vi "Value.vi"(7 "Variables":refnum<class "Variables.lvclass">, 11 "Condition Value in":refnum<class "Condition Value.lvclass">) -> (2 "error out":errorcluster, 3 "Value":dbl)   [LabVIEW 2020, in "VolatusSeq.lvlib" / "Condition Value.lvclass"]
uses:
  Condition Value.lvclass
  Variables/Variables.lvclass
  Condition Value.lvclass/Condition Value.ctl
  lv-vecto/Vecto/Channel DBL/Channel DBL.lvclass/Channel DBL.ctl
  Variables/Variables.lvclass/Variables.ctl
  lv-vecto/Vecto/Group DBL/Value by Index.vi
  lv-vecto/Vecto/Channel DBL/Channel DBL.lvclass
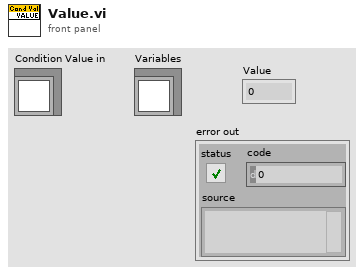
[diagram p1: front panel]
types:
  T1 = typedef "VolatusSeq.lvlib/Value Source.ctl" = enum16{"Channel", "Variable", "Expression"}
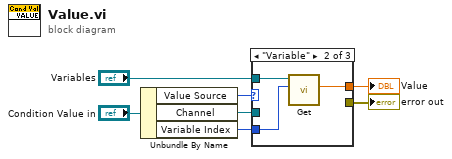
[diagram p0: block diagram]
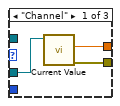
[diagram p2: hidden frame]
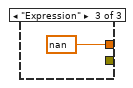
[diagram p3: hidden frame]
diagram:
  n1 = Unbundle By Name("Condition Value in") -> ("Value Source"=w5:T1, "Channel"=w6:refnum<class "Channel DBL.lvclass">, "Variable Index"=w4:i32)
  n2 = case shown="\"Variable\"" w5 {
    tunnel: w6 -> [w10 _ _]
    tunnel: w4 -> [_ w12 _]
    tunnel: "Variables" -> [_ w13 _]
    tunnel: [w9 w11 nan ("Value")] -> w2
    tunnel: [w8 _ _] -> w1
    frame "Channel" {
      n3 = call "Current Value.vi"("Channel in"=w10) -> ("error out"=w8:errorcluster, "Scaled"=w9:dbl)  [unwired: 6 in, 3 out]
    }
    frame "Variable" {
      n4 = call "Get.vi"("Index"=w12, "Variables in"=w13) -> ("Value"=w11:dbl)  [unwired: 9 in]
    }
    frame "Expression" {
    }
  }
  "Value" <- w2
  "error out" <- w1
